vi "_Build VIHLP path.vi"(0 "Documented VI path":path=path "C:/Projects/HELPer (LabVIEW Documentation Toolkit)/HELPer (versions)/HELPer 1.1.0.0/HELPer (VI Documentation Toolkit)/VI Documentation Tools/Add HTML Documentation for VI's parent item.vi", 11 "error in":errorcluster) -> (4 "Path to VIHLP file":path, 15 "error out":errorcluster)   [LabVIEW 2012]
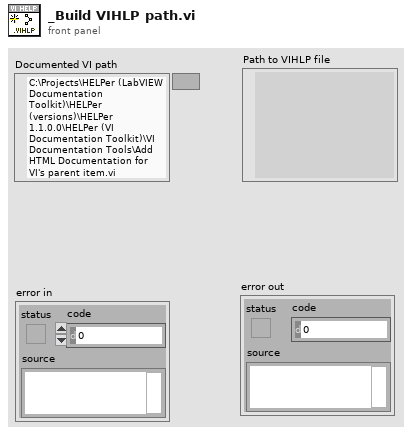
[diagram p1: front panel]
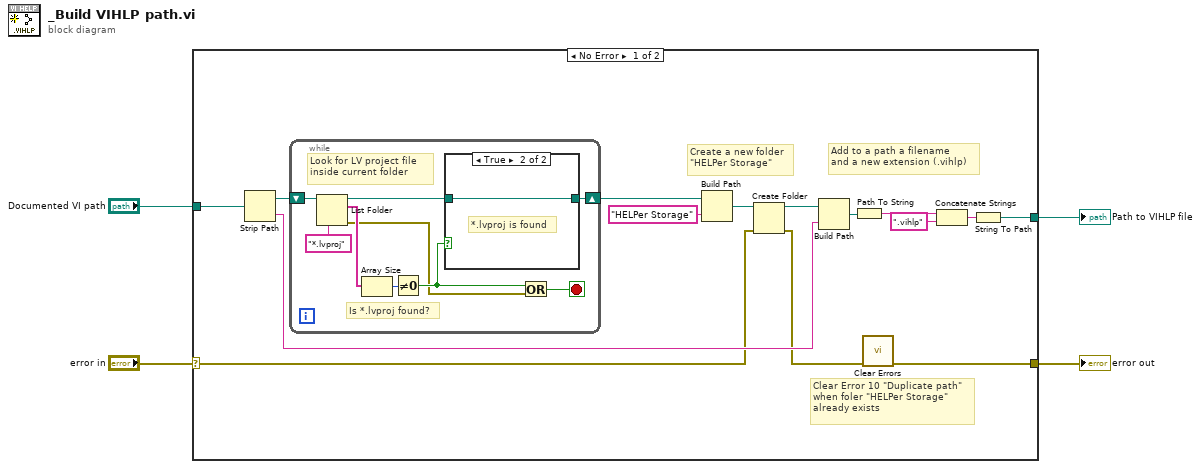
[diagram p0: block diagram]
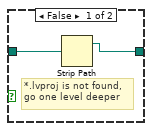
[diagram p2: hidden frame]
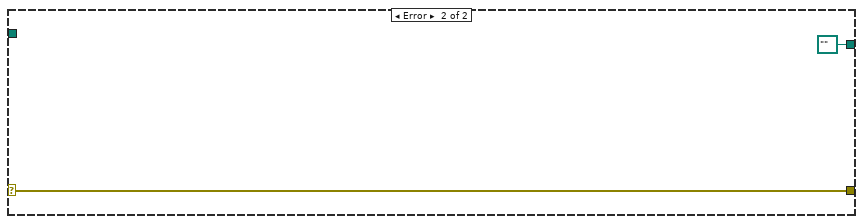
[diagram p3: hidden frame]
diagram:
  n1 = case shown="No Error" "error in" {
    selector: "error in" -> [w5 w33]
    tunnel: "Documented VI path" -> [w19 _]
    tunnel: [w8 path ""] -> w3
    tunnel: [w6 w33] -> w2
    frame No Error {
      # "Add to a path a filename\nand a new extension (.vihlp)"
      # "Create a new folder\n\"HELPer Storage\""
      # "Clear Error 10 \"Duplicate path\"\nwhen foler \"HELPer Storage\"\nalready exists"
      n2 = Strip Path(path=w19) -> (stripped path=w18:path, name=w9:string)
      n3 = while {
        shift-right: [w23] -> w17
        shift-left: w18 -> [w27]
        stop <- w21 stop-if-true
        # "Look for LV project file \ninside current folder"
        # "Is *.lvproj found?"
        n4 = List Folder(path=w27, pattern="*.lvproj") -> (path out=w24:path, filenames=w26:string[], error out=w20:errorcluster)  [unwired: 2 in, 1 out]
        n5 = Array Size(array=w26) -> (size(s)=w25:i32)
        n6 = Not Equal To 0?(x=w25) -> (x != 0?=w22:bool)
        n7 = case shown="True" w22 {
          tunnel: w24 -> [w30 w31]
          tunnel: [w29 w31] -> w23
          frame False {
            # "*.lvproj is not found,\ngo one level deeper"
            n8 = Strip Path(path=w30) -> (stripped path=w29:path)  [unwired: 1 out]
          }
          frame True {
            # "*.lvproj is found"
          }
        }
        n9 = Or(x=w22, y=w20) -> (x .or. y?=w21:bool)
      }
      n10 = Build Path(base path=w17, name or relative path="HELPer Storage") -> (appended path=w15:path)
      n11 = Create Folder(path (use dialog)=w15, error in=w5) -> (created path=w14:path, error out=w7:errorcluster)  [unwired: 1 in, 1 out]
      n12 = Build Path(base path=w14, name or relative path=w9) -> (appended path=w10:path)
      n13 = Path To String(path=w10) -> (string=w13:string)
      n14 = call <vilib>:"Clear Errors.vi"("error in (no error)"=w7) -> ("error out"=w6:errorcluster)  [unwired: 6 in]
      n15 = Concatenate Strings(w13, ".vihlp" ("string")) -> (w11:string)
      n16 = String To Path(string=w11) -> (path=w8:path)
    }
    frame Error {
    }
  }
  "Path to VIHLP file" <- w3
  "error out" <- w2
